vi "TOML-to-tree.vi"(5 "tag":string, 7 "name":string, 8 "error in":errorcluster, 9 "purge":bool caption="purge (True)", 10 "value":T1, 11 "tree-control-ref":refnum<vi>) -> (0 "error out":errorcluster)   [LabVIEW 2020, in "TOML.lvlib"]
uses:
  TOML.lvlib
  TOML Value.ctl
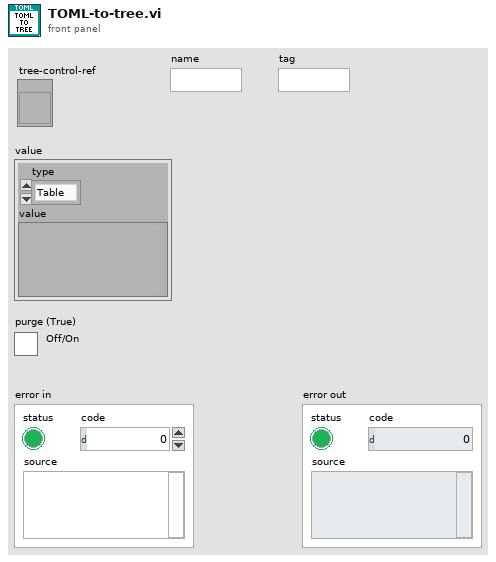
[diagram p1: front panel]
types:
  T1 = typedef "TOML.lvlib/TOML Value.ctl" = cluster{"type":enum16{"Table", "Array", "String", "Integer", "Float", "Boolean", "Offset Date-Time", "Local Date-Time", "Local Date", "Local Time", "Path"}, "value":variant}
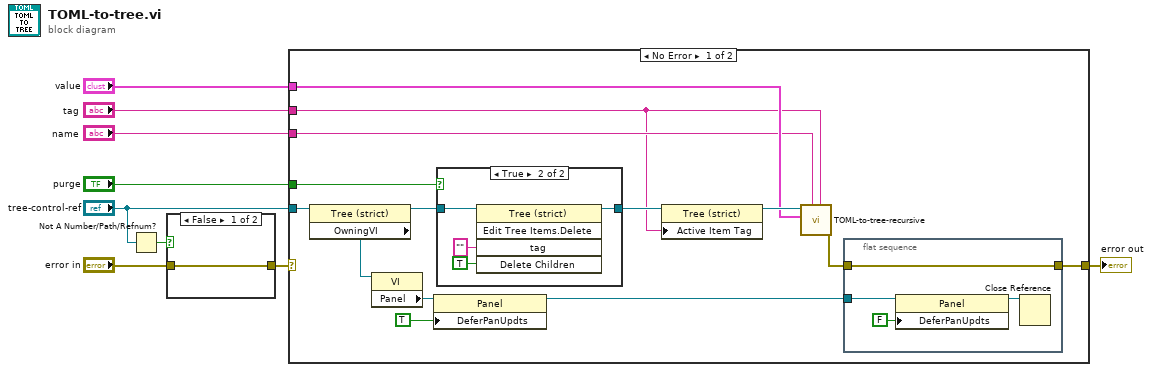
[diagram p0: block diagram]
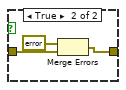
[diagram p2: hidden frame]
diagram:
  n1 = Not A Number/Path/Refnum?(number/path/refnum="tree-control-ref") -> (NaN/Path/Refnum?=w4:bool)
  n2 = case shown="False" w4 {
    tunnel: "error in" -> [w10 w12]
    tunnel: [w10 w13] -> w2
    frame False {
    }
    frame True {
      n3 = Merge Errors(errorcluster {"status"=TRUE, "code"=97, "source"="invalid tree reference"} ("error in"), w12) -> (w13:errorcluster)
    }
  }
  n4 = case shown="No Error" w2 {
    selector: w2 -> [_ w37]
    tunnel: "value" -> [w19 _]
    tunnel: "name" -> [w18 _]
    tunnel: "tree-control-ref" -> [w25 _]
    tunnel: "tag" -> [w17 _]
    tunnel: [w15 w37] -> w6
    tunnel: "purge" -> [w27 _]
    frame No Error {
      n5 = property class="Tree (strict)"(reference=w25) -> (reference out=w24:refnum<vi>, "OwningVI"=w23:refnum<vi>)  [unwired: 1 in, 1 out]
      n6 = property class="VI"(reference=w23) -> ("Panel"=w22:refnum<vi>)  [unwired: 1 in, 2 out]
      n7 = property class="Panel"(reference=w22, "DeferPanUpdts"=TRUE ("Defer Panel Updates")) -> (reference out=w16:refnum<vi>)  [unwired: 1 in, 1 out]
      n8 = case shown="True" w27 {
        tunnel: w24 -> [w32 w34]
        tunnel: [w32 w33] -> w26
        frame False {
        }
        frame True {
          n9 = invoke class="Tree (strict)" method="Edit Tree Items.Delete"(reference=w34, "tag"="" ("Tag"), "Delete Children"=TRUE ("Delete Children?")) -> (reference out=w33:refnum<vi>)  [unwired: 2 in, 4 out]
        }
      }
      n10 = property class="Tree (strict)"(reference=w26, "Active Item Tag"=w17) -> (reference out=w20:refnum<vi>)  [unwired: 1 in, 1 out]
      n11 = call "TOML-to-tree-recursive.vi"("tag"=w17, "name"=w18, "value"=w19, "tree-control-ref"=w20) -> ("error out"=w14:errorcluster)  [unwired: 7 in]
      n12 = flat-sequence {
        tunnel: w16 -> [w29]
        tunnel: [w28] -> w15
        tunnel: w14 -> [w28]
        frame #0 {
          n13 = property class="Panel"(reference=w29, "DeferPanUpdts"=FALSE ("Defer Panel Updates")) -> (reference out=w30:refnum<vi>)  [unwired: 1 in, 1 out]
          n14 = Close Reference(reference=w30) -> ()  [unwired: 1 in, 1 out]
        }
      }
    }
    frame Error {
    }
  }
  "error out" <- w6
